vi "ArrayList DEMO.vi"() -> ()   [LabVIEW 2012]
uses:
  ArrayList/ArrayListClass.lvclass
panel:
  out "错误输出":errorcluster
  out "数据":i32[](array[numeric])
  out "数据":i32[](array[numeric])
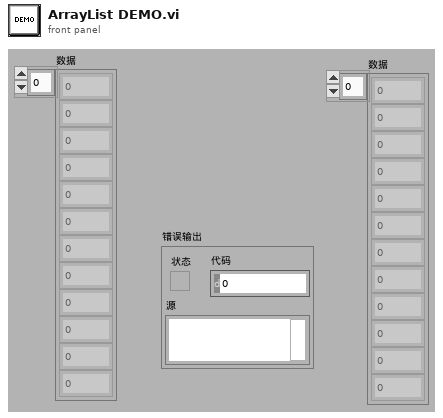
[diagram p1: front panel]
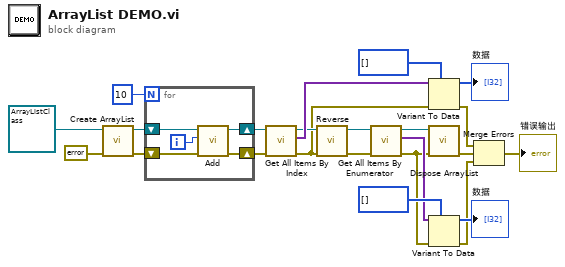
[diagram p0: block diagram]
diagram:
  n1 = call "Create ArrayList.vi"("error in (no error)"=errorcluster {"status"=FALSE, "code"=0, "source"=""}, "ArrayListClass 输入"=refnum<class "ArrayListClass.lvclass"> refnum ("ArrayListClass.lvclass")) -> ("error out"=w1:errorcluster, "ArrayListClass 输出"=w2:refnum<class "ArrayListClass.lvclass">)  [unwired: 8 in]
  n2 = for {
    N: 10 -> [_]
    shift-right: [w25] -> w17
    shift-left: w2 -> [w28]
    shift-right: [w26] -> w22
    shift-left: w1 -> [w27]
    i -> [w24]
    n3 = call "Add.vi"("error in (no error)"=w27, "anything"=w24, "ArrayListClass 输入"=w28) -> ("error out"=w26:errorcluster, "ArrayListClass 输出"=w25:refnum<class "ArrayListClass.lvclass">)  [unwired: 7 in]
  }
  n4 = call "Get All Items By Index.vi"("error in (no error)"=w22, "ArrayListClass 输入"=w17) -> ("error out"=w7:errorcluster, "Items"=w20:variant[], "ArrayListClass 输出"=w10:refnum<class "ArrayListClass.lvclass">)  [unwired: 7 in]
  n5 = call "Reverse.vi"("error in (no error)"=w7, "ArrayListClass 输入"=w10) -> ("error out"=w14:errorcluster, "ArrayListClass 输出"=w15:refnum<class "ArrayListClass.lvclass">)  [unwired: 8 in]
  n6 = call "Get All Items By Enumerator.vi"("error in (no error)"=w14, "ArrayListClass 输入"=w15) -> ("error out"=w8:errorcluster, "Items"=w11:variant[], "ArrayListClass 输出"=w9:refnum<class "ArrayListClass.lvclass">)  [unwired: 7 in]
  n7 = Variant To Data(error in=w7, type=i32[] [], Variant=w20) -> (data=→"数据":i32[], error out=w6:errorcluster)
  n8 = call "Dispose ArrayList.vi"("error in (no error)"=w8, "ArrayListClass 输入"=w9) -> ("error out"=w5:errorcluster)  [unwired: 8 in, 1 out]
  n9 = Variant To Data(error in=w8, type=i32[] [], Variant=w11) -> (data=→"数据":i32[], error out=w4:errorcluster)
  n10 = Merge Errors(w6, w5, w4) -> (→"错误输出":errorcluster)
